vi "Open.vi"(8 "error in (no error)":errorcluster, 11 "Shutter in":refnum<class "Shutter.lvclass">) -> (0 "error out":errorcluster, 3 "Shutter out":refnum<class "Shutter.lvclass">)   [LabVIEW 2016, in "Shutter.lvclass"]
uses:
  Shutter.lvclass
  Shutter.lvclass/Shutter.ctl
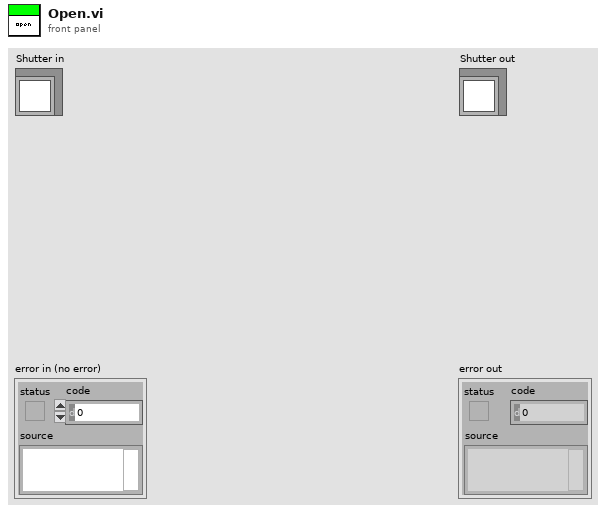
[diagram p1: front panel]
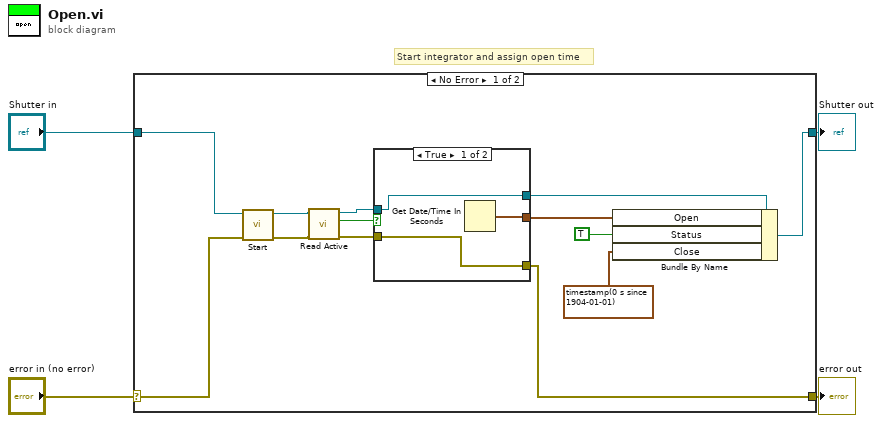
[diagram p0: block diagram]
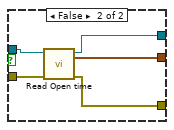
[diagram p2: hidden frame]
diagram:
  # "Start integrator and assign open time"
  n1 = case shown="No Error" "error in (no error)" {
    selector: "error in (no error)" -> [w17 w27]
    tunnel: [w6 w27] -> w3
    tunnel: [w8 w26] -> w1
    tunnel: "Shutter in" -> [w16 w26]
    frame No Error {
      n2 = call-dynamic "Start.vi"("error in (no error)"=w17, "Integrator in"=w16) -> ("error out"=w14:errorcluster, "Integrator out"=w15:refnum<class "Shutter.lvclass">)  [unwired: 8 in]
      n3 = call-dynamic "Read Active.vi"("error in (no error)"=w14, "Integrator in"=w15) -> ("error out"=w11:errorcluster, "Active"=w13:bool, "Integrator out"=w12:refnum<class "Shutter.lvclass">)  [unwired: 7 in]
      n4 = case shown="True" w13 {
        tunnel: w12 -> [w19 w25]
        tunnel: w11 -> [w18 w24]
        tunnel: [w20 w23] -> w9
        tunnel: [w19 w22] -> w7
        tunnel: [w18 w21] -> w6
        frame True {
          n5 = Get Date/Time In Seconds() -> (seconds since 1Jan1904=w20:timestamp)
        }
        frame False {
          n6 = call-dynamic "Read Open time.vi"("error in (no error)"=w24, "Integrator in"=w25) -> ("error out"=w21:errorcluster, "Open time"=w23:timestamp, "Integrator out"=w22:refnum<class "Shutter.lvclass">)  [unwired: 7 in]
        }
      }
      n7 = Bundle By Name(cluster=w7, "Open"=w9, "Status"=TRUE ("Shutter.Status"), "Close"=timestamp(0 s since 1904-01-01) ("Open")) -> (w8:refnum<class "Shutter.lvclass">)
    }
    frame Error {
    }
  }
  "error out" <- w3
  "Shutter out" <- w1
